vi "to_ustupidorogu.vi"() -> ()   [LabVIEW 2017]
uses:
  <vilib>/userdefined/High Color/IMAQdx.ctl
  <vilib>/vision/driver/NI_Vision_Acquisition_Software.lvlib
panel:
  out "X":sgl
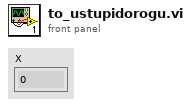
[diagram p1: front panel]
types:
  T1 = typedef "IMAQdx.ctl" = refnum<k21>
  T2 = typedef "IMAQ Image.ctl" = refnum<image>
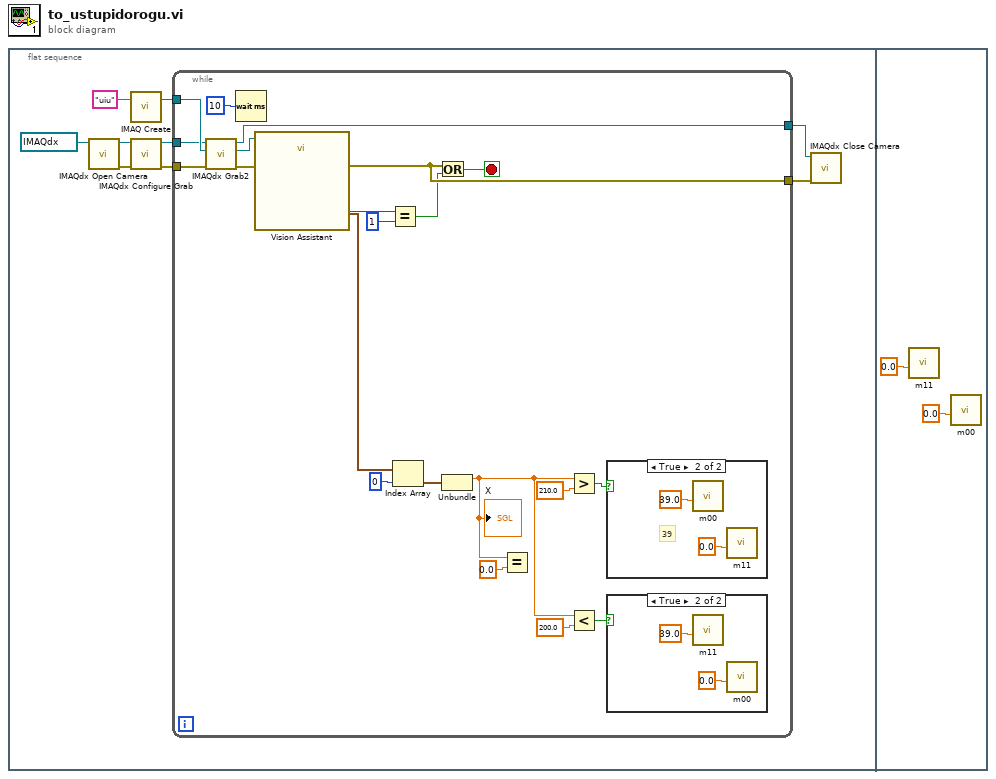
[diagram p0: block diagram]
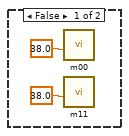
[diagram p2: hidden frame]
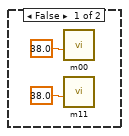
[diagram p3: hidden frame]
diagram:
  n1 = flat-sequence {
    frame #0 {
      n2 = call <vilib>:"IMAQdx Open Camera.vi"("Session In"=T1 "cam1") -> ("error out"=w6:errorcluster, "Session Out"=w5:T1)  [unwired: 9 in]
      n3 = call "IMAQ Create"("Image Name"="uiu") -> ("New Image"=w3:T2)  [unwired: 4 in, 1 out]
      n4 = call <vilib>:"IMAQdx Configure Grab.vi"("error in"=w6, "Session In"=w5) -> ("error out"=w7:errorcluster, "Session Out"=w4:T1)  [unwired: 8 in]
      n5 = while {
        tunnel: w7 -> [w25]
        tunnel: w3 -> [w24]
        tunnel: w4 -> [w23]
        tunnel: [w22] -> w9
        tunnel: [w20] -> w8
        stop <- w21 stop-if-true
        n6 = call <vilib>:"IMAQdx Grab2.vi"("error in"=w25, "Image In"=w24, "Session In"=w23) -> ("error out"=w27:errorcluster, "Image Out"=w26:T2, "Session Out"=w22:T1)  [unwired: 5 in, 1 out]
        n7 = Wait (ms)(milliseconds to wait=u32 10) -> ()  [unwired: 1 out]
        n8 = call "Vision Assistant"("Image In"=w26, "error in"=w27) -> ("Edges Coordinates (Edge Detector 1)"=w30:cluster{"X":sgl, "Y":sgl}[], "Number of Matches (Color Location 1)"=w12:i32, "error out"=w20:errorcluster)  [unwired: 22 in, 1 out]
        n9 = Equal?(x=w12, y=1) -> (x = y?=w11:bool)
        n10 = Index Array(array=w30, index=0) -> (element=w29:cluster{"X":sgl, "Y":sgl})
        n11 = Or(x=w20, y=w11) -> (x .or. y?=w21:bool)
        n12 = Unbundle(w29) -> ("X"=w15:sgl)  [unwired: 1 out]
        "X" <- w15
        n13 = Equal?(x=w15, y=sgl 0.0) -> ()  [unwired: 1 out]
        n14 = Greater?(x=w15, y=sgl 210.0) -> (0:w18:bool)
        n15 = Less?(x=w15, y=sgl 200.0) -> (x < y?=w14:bool)
        n16 = case shown="True" w18 {
          frame False {
            n17 = call "m00.vi"("position"=38.0) -> ()  [unwired: 10 in, 1 out]
            n18 = call "m11.vi"("position"=38.0) -> ()  [unwired: 10 in, 1 out]
          }
          frame True {
            # "39"
            n19 = call "m00.vi"("position"=39.0) -> ()  [unwired: 10 in, 1 out]
            n20 = call "m11.vi"("position"=0.0) -> ()  [unwired: 10 in, 1 out]
          }
        }
        n21 = case shown="True" w14 {
          frame False {
            n22 = call "m00.vi"("position"=38.0) -> ()  [unwired: 10 in, 1 out]
            n23 = call "m11.vi"("position"=38.0) -> ()  [unwired: 10 in, 1 out]
          }
          frame True {
            n24 = call "m11.vi"("position"=39.0) -> ()  [unwired: 10 in, 1 out]
            n25 = call "m00.vi"("position"=0.0) -> ()  [unwired: 10 in, 1 out]
          }
        }
      }
      n26 = call <vilib>:"IMAQdx Close Camera.vi"("error in"=w8, "Session In"=w9) -> ()  [unwired: 9 in, 1 out]
    }
    frame #1 {
      n27 = call "m11.vi"("position"=0.0) -> ()  [unwired: 10 in, 1 out]
      n28 = call "m00.vi"("position"=0.0) -> ()  [unwired: 10 in, 1 out]
    }
  }
